vi "DI Pulse Gen.vi"(0 "Channel Enable":bool, 1 "MAX_CAT":u16, 2 "Stroke (FALSE=2, TRUE=4)":bool=TRUE, 3 "Window_End (DBTDC)":sgl, 4 "Window_Start (DBTDC)":sgl, 5 "TDC (Absolute CAD)":sgl, 7 "InjPulseSwitchArray":bool[](array[boolean]), 9 "FuelTiming [DBTDC]":T1, 11 "FuelDuration[msec]":T2) -> (8 "PlsGen_Config_Out":T3)   [LabVIEW 2015, in "ECS-RT.lvlib"]
uses:
  ECS-RT.lvlib
  <vilib>/Powertrain Controls/Device Drivers/Tools/Real-Time/time2ticks.vi
  <vilib>/Powertrain Controls/Device Drivers/Tools/Real-Time/Offset2CAT.vi
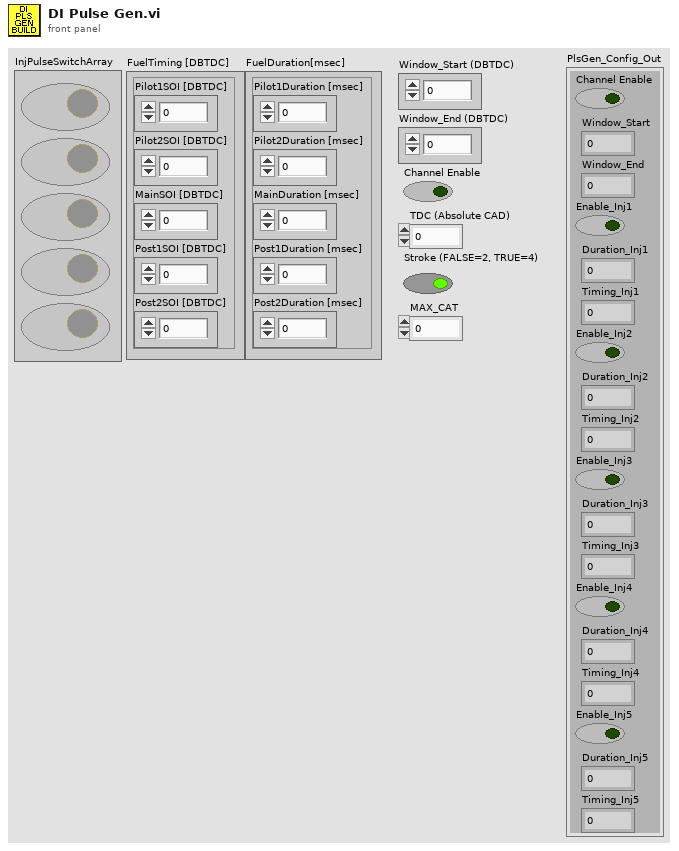
[diagram p1: front panel]
types:
  T1 = cluster{"Pilot1SOI [DBTDC]":sgl, "Pilot2SOI [DBTDC]":sgl, "MainSOI [DBTDC]":sgl, "Post1SOI [DBTDC]":sgl, "Post2SOI [DBTDC]":sgl}
  T2 = cluster{"Pilot1Duration [msec]":sgl, "Pilot2Duration [msec]":sgl, "MainDuration [msec]":sgl, "Post1Duration [msec]":sgl, "Post2Duration [msec]":sgl}
  T3 = cluster{"Channel Enable":bool, "Window_Start":u16, "Window_End":u16, "Enable_Inj1":bool, "Duration_Inj1":u32, "Timing_Inj1":u16, "Enable_Inj2":bool, "Duration_Inj2":u32, "Timing_Inj2":u16, "Enable_Inj3":bool, "Duration_Inj3":u32, "Timing_Inj3":u16, "Enable_Inj4":bool, "Duration_Inj4":u32, "Timing_Inj4":u16, "Enable_Inj5":bool, "Duration_Inj5":u32, "Timing_Inj5":u16}
  T4 = cluster{"Window_Start (DBTDC)":sgl, "Window_End (DBTDC)":sgl, "Enable_Inj1":bool, "Duration_Inj1 (msec)":sgl, "Timing_Inj1 (DBTDC)":sgl, "Enable_Inj2":bool, "Duration_Inj2 (msec)":sgl, "Timing_Inj2 (DBTDC)":sgl, "Enable_Inj3":bool, "Duration_Inj3 (msec)":sgl, "Timing_Inj3 (DBTDC)":sgl, "Enable_Inj4":bool, "Duration_Inj4 (msec)":sgl, "Timing_Inj4 (DBTDC)":sgl, "Enable_Inj5":bool, "Duration_Inj5 (msec)":sgl, "Timing_Inj5 (DBTDC)":sgl}
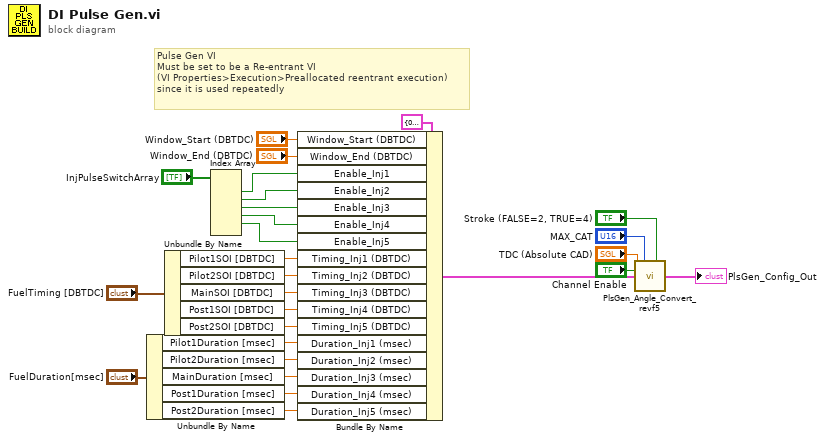
[diagram p0: block diagram]
diagram:
  # "Pulse Gen VI\nMust be set to be a Re-entrant VI \n(VI Properties>Execution>Preallocated reentrant execution)\nsince it is used repeatedly"
  n1 = Unbundle By Name("FuelDuration[msec]") -> ("Pilot1Duration [msec]"=w6:sgl, "Pilot2Duration [msec]"=w4:sgl, "MainDuration [msec]"=w3:sgl, "Post1Duration [msec]"=w2:sgl, "Post2Duration [msec]"=w1:sgl)
  n2 = Unbundle By Name("FuelTiming [DBTDC]") -> ("Pilot1SOI [DBTDC]"=w11:sgl, "Pilot2SOI [DBTDC]"=w10:sgl, "MainSOI [DBTDC]"=w9:sgl, "Post1SOI [DBTDC]"=w8:sgl, "Post2SOI [DBTDC]"=w7:sgl)
  n3 = Index Array(array="InjPulseSwitchArray") -> (element #1=w17:bool, element #2=w16:bool, element #3=w15:bool, element #4=w14:bool, element #5=w13:bool)  [unwired: 6 in, 1 out]
  n4 = Bundle By Name(cluster=T4 {"Window_Start (DBTDC)"=0.0, "Window_End (DBTDC)"=0.0, "Enable_Inj1"=FALSE, "Duration_Inj1 (msec)"=0.0, "Timing_Inj1 (DBTDC)"=0.0, "Enable_Inj2"=FALSE, "Duration_Inj2 (msec)"=0.0, "Timing_Inj2 (DBTDC)"=0.0, "Enable_Inj3"=FALSE, "Duration_Inj3 (msec)"=0.0, "Timing_Inj3 (DBTDC)"=0.0, "Enable_Inj4"=FALSE, "Duration_Inj4 (msec)"=0.0, "Timing_Inj4 (DBTDC)"=0.0, "Enable_Inj5"=FALSE, "Duration_Inj5 (msec)"=0.0, "Timing_Inj5 (DBTDC)"=0.0} ("PlsGen_Angle_Config_In"), "Window_Start (DBTDC)"="Window_Start (DBTDC)", "Window_End (DBTDC)"="Window_End (DBTDC)", "Enable_Inj1"=w17, "Enable_Inj2"=w16, "Enable_Inj3"=w15, "Enable_Inj4"=w14, "Enable_Inj5"=w13, "Timing_Inj1 (DBTDC)"=w11, "Timing_Inj2 (DBTDC)"=w10, "Timing_Inj3 (DBTDC)"=w9, "Timing_Inj4 (DBTDC)"=w8, "Timing_Inj5 (DBTDC)"=w7, "Duration_Inj1 (msec)"=w6, "Duration_Inj2 (msec)"=w4, "Duration_Inj3 (msec)"=w3, "Duration_Inj4 (msec)"=w2, "Duration_Inj5 (msec)"=w1) -> (w27:T4)
  n5 = call <vilib>:"PlsGen_Angle_Convert_revf5.vi"("TDC (Absolute CAD)"="TDC (Absolute CAD)", "MAX_CAT"="MAX_CAT", "Stroke (FALSE=2, TRUE=4)"="Stroke (FALSE=2, TRUE=4)", "Channel Enable"="Channel Enable", "PlsGen_Angle_Config_In"=w27) -> ("PlsGen_Config_Out"=→"PlsGen_Config_Out":T3)  [unwired: 10 in]
